vi "CRYCorrect Frequency and Step.vi"(4 "Steps":u32, 6 "Resolution":u16, 8 "Stop Frequency":dbl=100.0, 9 "Start Frequency":dbl=1.0, 10 "Sampling Rate":dbl=1.0, 11 "Sweep type":i32) -> (1 "Steps":u32, 2 "Stop Freq Out":dbl, 3 "Start Freq Out":dbl)   [LabVIEW 2013]
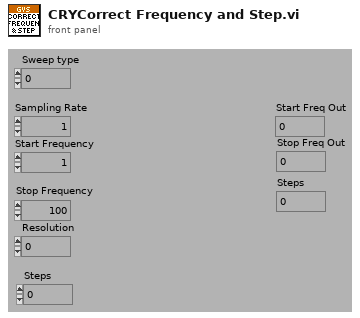
[diagram p1: front panel]
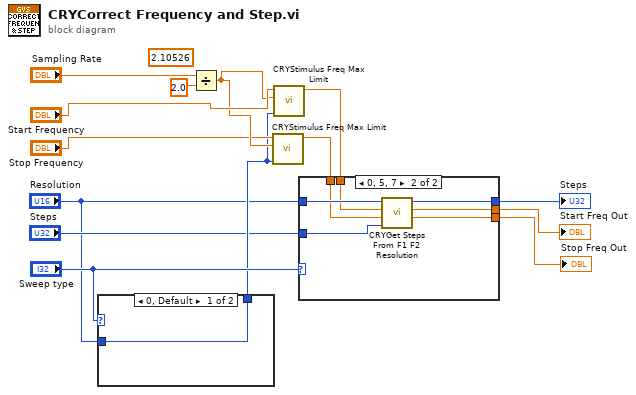
[diagram p0: block diagram]
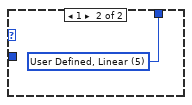
[diagram p2: hidden frame]
diagram:
  (unwired) 2.10526 ("y")
  n1 = case shown="0, Default" "Sweep type" {
    tunnel: [w15 w16] -> w3
    tunnel: "Resolution" -> [w15 _]
    frame 0, Default {
    }
    frame 1 {
      w16 = u16 5 items=["R10 (1/3 Oct.)", "R20 (1/6 Oct.)", "R40 (1/12 Oct.)", "R80 (1/24 Oct.)", "User Defined, Log", "User Defined, Linear"] ("Step size")
    }
  }
  n2 = Divide(x="Sampling Rate", y=2.0) -> (x/y=w8:dbl)
  n3 = call "CRYStimulus Freq Max Limit.vi"("Resolution"=w3, "Max Freq"=w8, "Input Val"="Stop Frequency") -> ("Output Val"=w5:dbl)  [unwired: 1 in, 7 out]
  n4 = call "CRYStimulus Freq Max Limit.vi"("Resolution"=w3, "Max Freq"=w8, "Input Val"="Start Frequency") -> ("Output Val"=w6:dbl)  [unwired: 1 in, 7 out]
  n5 = case shown="0, 5, 7" "Sweep type" {
    tunnel: "Steps" -> [w19 w20]
    tunnel: [w19 w25] -> w13
    tunnel: "Resolution" -> [_ w26]
    tunnel: [w18 w24] -> w11
    tunnel: [w17 w23] -> w10
    tunnel: w6 -> [w18 w22]
    tunnel: w5 -> [w17 w21]
    frame Default {
    }
    frame 0, 5, 7 {
      n6 = call "CRYGet Steps From F1 F2 Resolution.vi"("Steps/Tone"=w20, "Stop Freq"=w21, "Start Freq"=w22, "Resolution"=w26) -> ("Stop Freq Out"=w23:dbl, "Start Freq Out"=w24:dbl, "Steps"=w25:i32)  [unwired: 5 out]
    }
  }
  "Steps" <- w13
  "Start Freq Out" <- w11
  "Stop Freq Out" <- w10
